vi "labvıew proje ödevi2.vi"() -> ()   [LabVIEW 2017]
uses:
  QR Code Generator v1.1.llb/User Option.ctl
  QR Code Generator v1.1.llb/EC Level.ctl
  <vilib>/Utility/miscctls.llb/LVBoundsTypeDef.ctl
  <vilib>/picture/picture.llb/Draw 1-Bit Pixmap.vi
panel:
  in  "Color":cluster{"Background":u32, "Foreground":u32}={"Background"=16777215, "Foreground"=0}
  in  "Image Size":u32=200 format="%.0d x %.0d pixels"
  out "Message":string
  in  "Save Button":bool
  in  "Directory name":path
  in  "Filename":string
  in  "Save image as":enum16{"JPG", "PNG", "BMP"}(ring)
  out "Preview:":picture
  in  "Error correction level:":T1
  in  "User Message":string caption="Please insert your message here:"
  in  "Stop Button":bool
  in  "User Options":T2 caption="Select the following options"
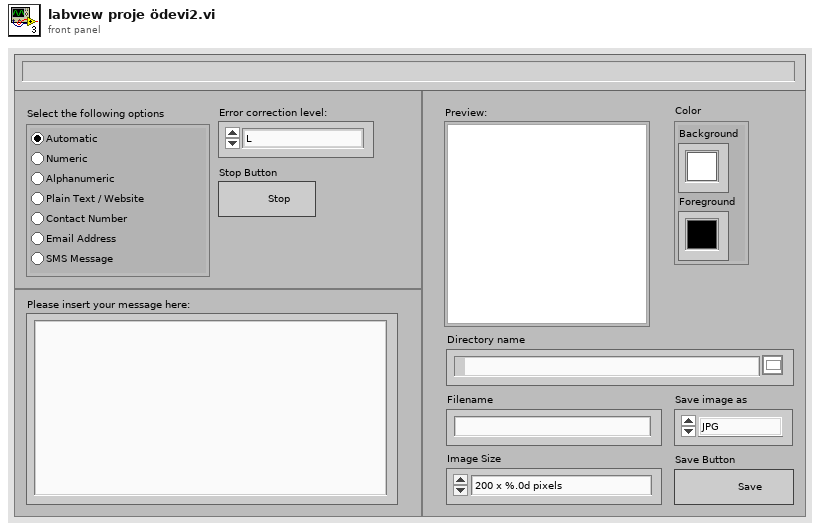
[diagram p1: front panel]
types:
  T1 = typedef "EC Level.ctl" = enum16{"L", "M", "Q", "H"}
  T2 = typedef "User Option.ctl" = enum32{"Automatic", "Numeric", "Alphanumeric", "Plain Text / Website", "Contact Number", "Email Address", "SMS Message"}
  T3 = typedef "LVBoundsTypeDef.ctl" = cluster{"Width":u32, "Height":u32}
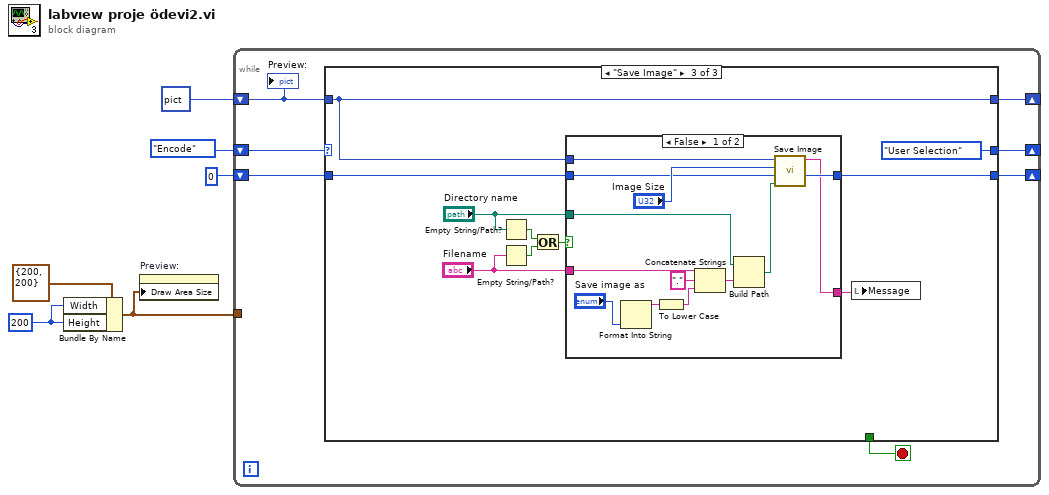
[diagram p0: block diagram]
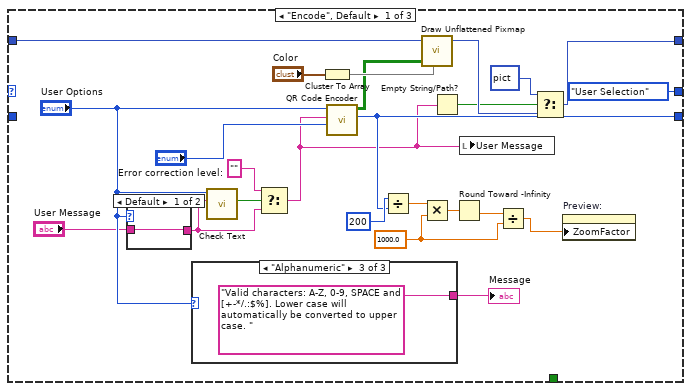
[diagram p2: hidden frame]
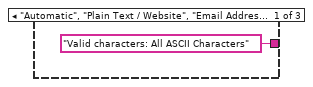
[diagram p3: hidden frame]
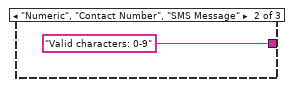
[diagram p4: hidden frame]
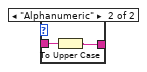
[diagram p5: hidden frame]
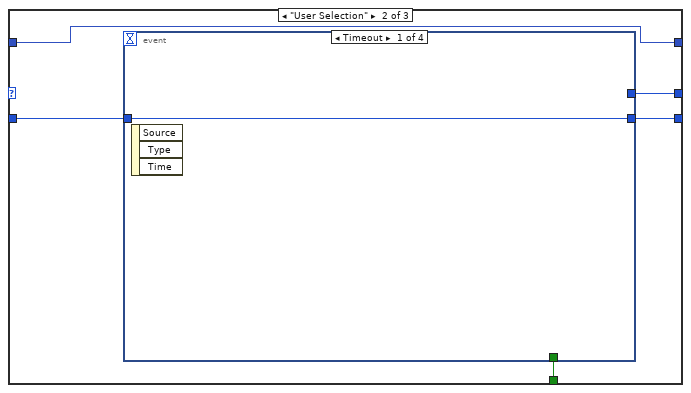
[diagram p6: hidden frame]
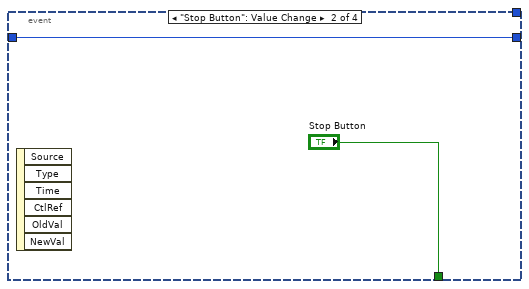
[diagram p7: hidden frame]
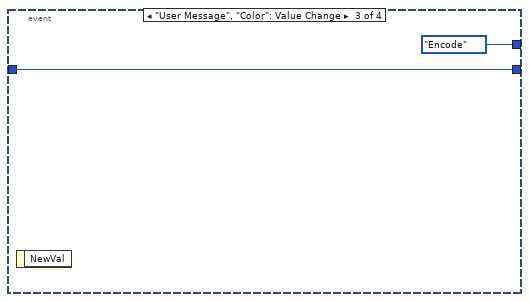
[diagram p8: hidden frame]
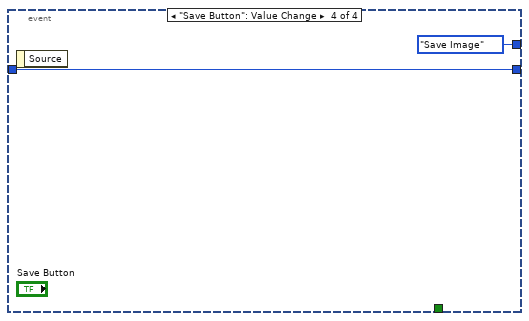
[diagram p9: hidden frame]
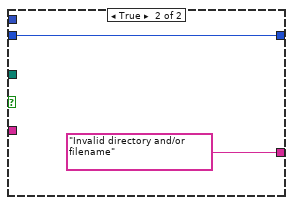
[diagram p10: hidden frame]
diagram:
  w3 = u32 200 ("Height")
  n1 = Bundle By Name(cluster=T3 {"Width"=200, "Height"=200} ("Draw Area Size"), "Width"=w3, "Height"=w3) -> (w2:T3)
  n2 = property on="Preview:" class="Pict"("Draw Area Size"=w2) -> ()  [unwired: 2 in, 2 out]
  n3 = while {
    shift-right: [w9] -> _
    shift-left: enum16{"Encode", "User Selection", "Save Image"}."Encode" -> [w13]
    shift-right: [w11] -> _
    shift-left: picture data[5B] ("new picture") -> [w12]
    tunnel: w2 -> [_]
    shift-right: [w10] -> _
    shift-left: 0 ("QR Size") -> [w8]
    stop <- w7 stop-if-true
    n4 = case shown="\"Save Image\"" w13 {
      tunnel: w12 -> [w26 w44 w56]
      tunnel: [w25 w44 w56] -> w11
      tunnel: [w24 w47 w57] -> w10
      tunnel: [enum16{"Encode", "User Selection", "Save Image"}."User Selection" w45 enum16{"Encode", "User Selection", "Save Image"}."User Selection"] -> w9
      tunnel: w8 -> [_ w48 w58]
      tunnel: [_ w46 _] -> w7
      frame "Encode", Default {
        w15 = 1000.0 ("y")
        n5 = case shown="Default" "User Options" {
          tunnel: "User Message" -> [w41 w43]
          tunnel: [w41 w42] -> w37
          frame Default {
          }
          frame "Alphanumeric" {
            n6 = To Upper Case(1:w43) -> (0:w42:string)
          }
        }
        n7 = case shown="\"Alphanumeric\"" "User Options" {
          tunnel: ["Valid characters: All ASCII Characters" ("Please insert your message here:") "Valid characters: 0-9" ("Please insert your message here:") "Valid characters: A-Z, 0-9, SPACE and [+-*/.:$%]. Lower case will automatically be converted to upper case. " ("Please insert your message here:")] -> w22
          frame "Automatic", "Plain Text / Website", "Email Address", Default {
          }
          frame "Numeric", "Contact Number", "SMS Message" {
          }
          frame "Alphanumeric" {
          }
        }
        "Message" <- w22
        n8 = call "Check Text.vi"("String"=w37, "Select the following options"="User Options") -> ("Invalid?"=w35:bool)  [unwired: 9 in]
        n9 = Select(t="", s=w35, f=w37) -> (s? t:f=w23:string)
        n10 = Cluster To Array(cluster="Color") -> (array=w34:u32[])
        n11 = call "QR Code Encoder.vi"("EC Level"="Error correction level:", "Message"=w23, "User Option"="User Options") -> ("QR Size"=w24:i32, "QR Data"=w31:bool[][])  [unwired: 7 in]
        n12 = Divide(x=200, y=w24) -> (x/y=w18:dbl)
        n13 = call-poly <vilib>:"Draw Unflattened Pixmap.vi"("picture"=w26, "data"=w31, "color table"=w34) -> ("new picture"=w32:picture)  [unwired: 6 in]
        n14 = Multiply(x=w18, y=w15) -> (x*y=w17:dbl)
        n15 = Empty String/Path?(string/path=w23) -> (empty?=w29:bool)
        n16 = Round Toward -Infinity(1:w17) -> (0:w16:dbl)
        n17 = local write "User Message"(w23) -> ()
        n18 = Divide(x=w16, y=w15) -> (x/y=w14:dbl)
        n19 = Select(t=picture data[5B], s=w29, f=w32) -> (s? t:f=w25:picture)
        n20 = property on="Preview:" class="Pict"("ZoomFactor"=w14) -> ()  [unwired: 2 in, 2 out]
      }
      frame "User Selection" {
        n21 = event shown="[0] Timeout" {
          selector: _ -> [_ _ _ _]
          dyn-events: _ -> [_ _ _ _]
          timeout: _ -> [_ _ _ _]
          tunnel: [_ "Stop Button" _ _] -> w46
          tunnel: w48 -> [w49 w50 w53 w55]
          tunnel: [w49 w50 w53 w55] -> w47
          tunnel: [_ _ enum16{"Encode", "User Selection", "Save Image"}."Encode" enum16{"Encode", "User Selection", "Save Image"}."Save Image"] -> w45
          event Timeout {
            n22 = event-data() -> ()  [unwired: 1 in, 3 out]
          }
          event "Stop Button": Value Change {
            n23 = event-data() -> ()  [unwired: 1 in, 6 out]
          }
          event "User Message", "Color": Value Change {
            n24 = event-data() -> ()  [unwired: 1 in, 1 out]
          }
          event "Save Button": Value Change {
            n25 = event-data() -> ()  [unwired: 1 in, 1 out]
          }
        }
      }
      frame "Save Image" {
        n26 = Empty String/Path?(string/path="Directory name") -> (empty?=w63:bool)
        n27 = Empty String/Path?(string/path="Filename") -> (empty?=w65:bool)
        n28 = Or(x=w63, y=w65) -> (x .or. y?=w64:bool)
        n29 = case shown="False" w64 {
          tunnel: [w67 "Invalid directory and/or filename" ("Please insert your message here:")] -> w60
          tunnel: "Directory name" -> [w68 _]
          tunnel: "Filename" -> [w73 _]
          tunnel: w56 -> [w71 _]
          tunnel: w58 -> [w69 w78]
          tunnel: [w69 w78] -> w57
          frame False {
            n30 = Format Into String("Save image as") -> (resulting string=w77:string)  [unwired: 3 in, 1 out]
            n31 = To Lower Case(string=w77) -> (all lower case string=w75:string)
            n32 = Concatenate Strings(w73, "." ("string"), w75) -> (w74:string)
            n33 = Build Path(base path=w68, name or relative path=w74) -> (appended path=w66:path)
            n34 = call "Save Image.vi"("Filepath"=w66, "QR Size"=w69, "Image Size"="Image Size", "2D Picture"=w71) -> ("Message"=w67:string)  [unwired: 7 in]
          }
          frame True {
          }
        }
        n35 = local write "Message"(w60) -> ()
      }
    }
    "Preview:" <- w12
  }
